vi "Execute Cycle Test.vi"(8 "error in (no error)":errorcluster, 10 "Action Data":variant, 11 "Controller in":refnum<class "Controller.lvclass">) -> (0 "error out":errorcluster, 3 "Controller out":refnum<class "Controller.lvclass">)   [LabVIEW 2020, in "Controller.lvlib" / "Controller.lvclass"]
uses:
  Controller.lvclass
  DataPool/ResArray.ctl
  Controller.lvclass/Controller.ctl
  Actor_log/Actor_log Messages/Write Event to Log Msg/Write Event to Log Msg.lvclass/Write Event to Log Msg.ctl
  <vilib>/ActorFramework/Message Enqueuer/Message Enqueuer.lvclass/Message Enqueuer.ctl
  Main_UI/Main_UI Messages/Update Cycle States Msg/Update Cycle States Msg.lvclass/Update Cycle States Msg.ctl
  Actor_AFG/Actor_AFG Messages/AFG Wait for Complete Msg/AFG Wait for Complete Msg.lvclass/AFG Wait for Complete Msg.ctl
  <vilib>/ActorFramework/Message Enqueuer/Enqueue.vi
  Actor_log/Actor_log Messages/Write Event to Log Msg/Write Event to Log Msg.lvclass
  C:/Program Files/National Instruments/LabVIEW 2020/vi.lib/ActorFramework/Message/Message.lvclass
  Main_UI/Main_UI Messages/Update Cycle States Msg/Update Cycle States Msg.lvclass
  Actor_AFG/Actor_AFG Messages/AFG Wait for Complete Msg/AFG Wait for Complete Msg.lvclass
  <vilib>/ActorFramework/Message Priority Queue/Priority Enqueue.vi
  DataPool/DataPool.lvlib
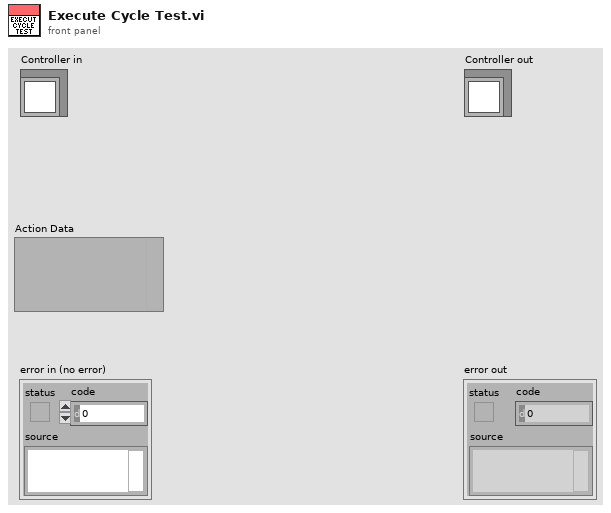
[diagram p1: front panel]
types:
  T1 = cluster{"Set Pulse Conf":cluster{"V Conf":cluster{"Bias":dbl, "Amp":dbl}, "T Conf":cluster{"Rise Time":dbl, "Fall Time":dbl, "Pulse Width":dbl}}, "Reset Pulse Conf":cluster{"V Conf":cluster{"Bias":dbl, "Amp":dbl}, "T Conf":cluster{"Rise Time":dbl, "Fall Time":dbl, "Pulse Width":dbl}}, "Cycle Timing":cluster{"Delay":dbl, "Pulse Spacing":dbl, "Burst Counts:":dbl, "Read Counts:":dbl}, "Read Voltage Setting":dbl}
  T2 = typedef "DataPool.lvlib/ResArray.ctl" = cluster{"Time":dbl, "Res":dbl}[]
  T3 = enum16{"Single Pulse", "Cycle_Idle", "Cycle_Running", "Cycle_Pause"}
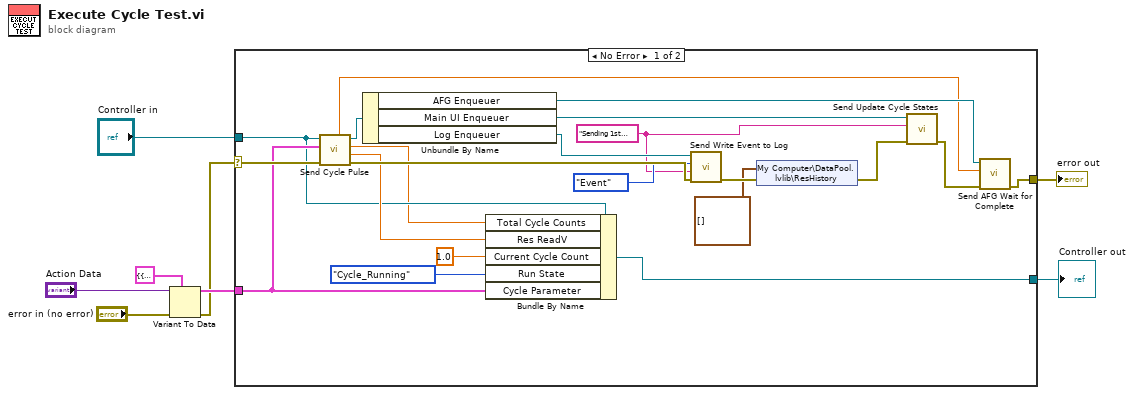
[diagram p0: block diagram]
diagram:
  n1 = Variant To Data(error in="error in (no error)", type=T1 {"Set Pulse Conf"={"V Conf"={"Bias"=1.0, "Amp"=2.5}, "T Conf"={"Rise Time"=5.0, "Fall Time"=5.0, "Pulse Width"=20.0}}, "Reset Pulse Conf"={"V Conf"={"Bias"=-0.5, "Amp"=-2.5}, "T Conf"={"Rise Time"=5.0, "Fall Time"=5.0, "Pulse Width"=20.0}}, "Cycle Timing"={"Delay"=0.0, "Pulse Spacing"=1.0, "Burst Counts:"=10.0, "Read Counts:"=1.0}, "Read Voltage Setting"=0.0}, Variant="Action Data") -> (data=w2:T1, error out=w1:errorcluster)
  n2 = case shown="No Error" w1 {
    selector: w1 -> [w29 w31]
    tunnel: [w9 w31] -> w8
    tunnel: [w24 w30] -> w6
    tunnel: "Controller in" -> [w19 w30]
    tunnel: w2 -> [w20 _]
    frame No Error {
      w13 = "Sending 1st Pulse sequence" ("Log Event Details")
      n3 = call "Send Cycle Pulse.vi"("error in (no error)"=w29, "Pulse Parameter"=w20, "Controller in"=w19) -> ("error out"=w28:errorcluster, "Read Voltage Setting"=w23:dbl, "Read Counts:"=w16:dbl, "Controller Out"=w17:refnum<class "Controller.lvclass">, "Time Before OPC?"=w11:dbl)  [unwired: 4 in]
      n4 = Unbundle By Name(w17) -> ("AFG Enqueuer"=w12:refnum<class "Message Enqueuer.lvclass">, "Main UI Enqueuer"=w15:refnum<class "Message Enqueuer.lvclass">, "Log Enqueuer"=w18:refnum<class "Message Enqueuer.lvclass">)
      n5 = Bundle By Name(cluster=w19, "Total Cycle Counts"=w16, "Res ReadV"=w23, "Current Cycle Count"=1.0, "Run State"=T3."Cycle_Running", "Cycle Parameter"=w20) -> (w24:refnum<class "Controller.lvclass">)
      n6 = call "Send Write Event to Log.vi"("error in (no error)"=w28, "Log Event Details"=w13, "Enum"=enum16{"Event", "Error"}."Event", "Message Enqueuer"=w18) -> ("error out"=w22:errorcluster)  [unwired: 6 in, 1 out]
      n7 = shared-variable "My Computer\\DataPool.lvlib\\ResHistory"(T2 [] ("ResHistory"), error in=w22) -> (error out=w14:errorcluster)
      n8 = call "Send Update Cycle States.vi"("error in (no error)"=w14, "Cycle State Message"=w13, "Message Enqueuer"=w15) -> ("error out"=w10:errorcluster)  [unwired: 7 in, 1 out]
      n9 = call "Send AFG Wait for Complete.vi"("error in (no error)"=w10, "Delay"=w11, "Message Enqueuer"=w12) -> ("error out"=w9:errorcluster)  [unwired: 7 in, 1 out]
    }
    frame Error {
    }
  }
  "error out" <- w8
  "Controller out" <- w6
